vi "Client Destroy.vi"(8 "error in (no error)":errorcluster, 11 "Telegram Class in":refnum<class "Telegram Class.lvclass">) -> (0 "error out":errorcluster, 3 "Telegram Class out":refnum<class "Telegram Class.lvclass">)   [LabVIEW 2015, in "Telegram Library.lvlib" / "Telegram Class.lvclass"]
doc: "Created IvanLis by LabVIEW Portal\nProfile: http://labviewportal.org/memberlist.php?mode=viewprofile&u=987\neMail: IvanLisanov@gMail.com\nTelegram: https://t.me/IvanLis"
uses:
  Telegram Class.lvclass
  Telegram Class.lvclass/Telegram Class.ctl
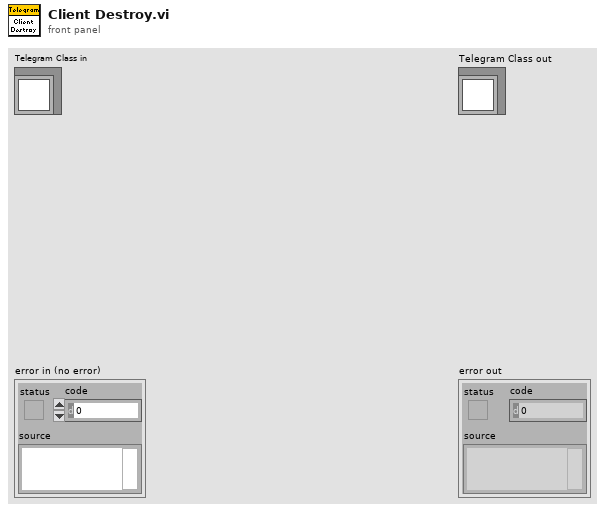
[diagram p1: front panel]
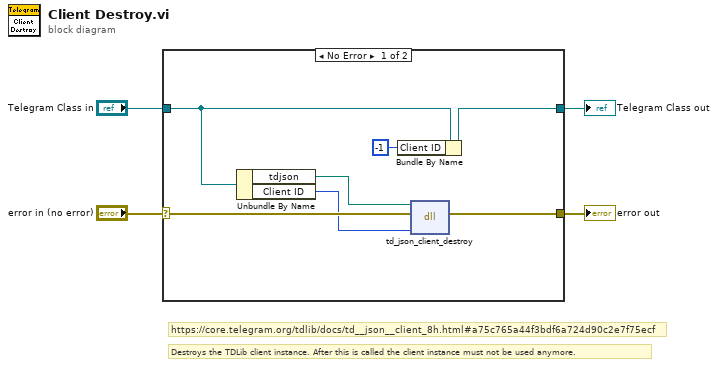
[diagram p0: block diagram]
diagram:
  # "Destroys the TDLib client instance. After this is called the client instance must not be used anymore."
  # "https://core.telegram.org/tdlib/docs/td__json__client_8h.html#a75c765a44f3bdf6a724d90c2e7f75ecf"
  n1 = case shown="No Error" "error in (no error)" {
    selector: "error in (no error)" -> [w8 w13]
    tunnel: [w6 w13] -> w3
    tunnel: [w10 w12] -> w1
    tunnel: "Telegram Class in" -> [w11 w12]
    frame No Error {
      n2 = Unbundle By Name(w11) -> ("tdjson"=w7:path, "Client ID"=w5:i32)
      n3 = Bundle By Name(cluster=w11, "Client ID"=-1) -> (w10:refnum<class "Telegram Class.lvclass">)
      n4 = dll-call lib="C:/Users/Ivan/Desktop/Telegram/Project/DLL/tdjson-x32.dll" fn="td_json_client_destroy"(path in=w7, error in=w8, "Client ID"=w5) -> (error out=w6:errorcluster)  [unwired: 3 in, 1 out]
    }
    frame Error {
    }
  }
  "error out" <- w3
  "Telegram Class out" <- w1
